vi "ENACreateMeas.vi"(0 "Meas in":T1={"S11"=TRUE, "S12"=TRUE, "S21"=TRUE, "S22"=TRUE}) -> (1 "Meas parameters":u16[](array[ring]) items=["S11", "S21", "S31", "S41", "S12", "S22", "S32", "S42", "S13", "S23", "S33", "S43", "S14", "S24", "S34", "S44", "A", "B", "C", "D", "R1", "R2", "R3", "R4", "AUX1", "AUX2", "TR", "T", "R"], 2 "Data format":u16[](array[ring]) items=["Logarithmic Magnitude", "Phase", "Group Delay", "Smith Chart  Linear (Lin/Phase)", "Smith Chart  Logarithmic (Log/Phase)", "Smith Chart  Complex (Real/Imag)", "Smith Chart  Impedance (R+jX)", "Smith Chart  Admittance (G+jB)", "Polar Format (Linear)", "Polar Format (Logarithmic)", "Polar Format (Re/Im)", "Linear Magnitude", "SWR", "Real", "Imaginary", "Epanded Phase", "Positive Phase"], 3 "Active trace":i32[](array[numeric]))   [LabVIEW 2017]
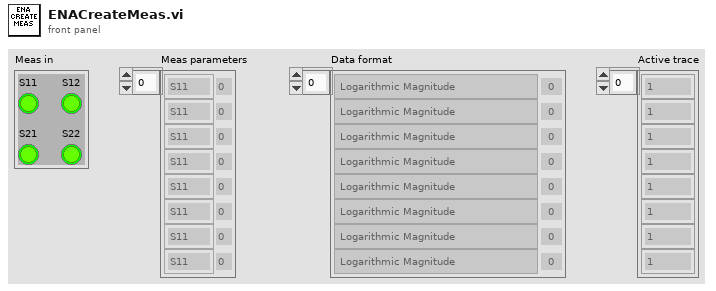
[diagram p1: front panel]
types:
  T1 = cluster{"S11":bool, "S12":bool, "S21":bool, "S22":bool}
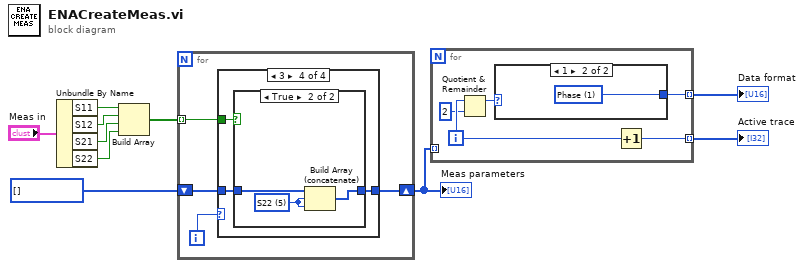
[diagram p0: block diagram]
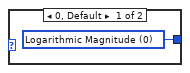
[diagram p2: hidden frame]
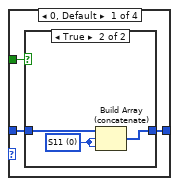
[diagram p3: hidden frame]
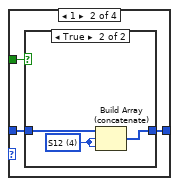
[diagram p5: hidden frame]
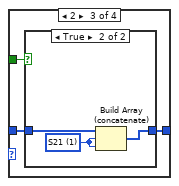
[diagram p7: hidden frame]
diagram:
  w4 = u16[] [] items=["S11", "S21", "S31", "S41", "S12", "S22", "S32", "S42", "S13", "S23", "S33", "S43", "S14", "S24", "S34", "S44", "A", "B", "C", "D", "R1", "R2", "R3", "R4", "AUX1", "AUX2", "TR", "T", "R"] ("Meas parameters 2")
  n1 = Unbundle By Name("Meas in") -> ("S11"=w9:bool, "S12"=w8:bool, "S21"=w7:bool, "S22"=w6:bool)
  n2 = Build Array(w9, w8, w7, w6) -> (w5:bool[])
  n3 = for {
    tunnel: w5 -> [w14] mode=indexing
    shift-right: [w11] -> w3
    shift-left: w4 -> [w13]
    i -> [w12]
    n4 = case shown="3" w12 {
      tunnel: w14 -> [w17 w24 w31 w38]
      tunnel: w13 -> [w16 w23 w30 w37]
      tunnel: [w15 w22 w29 w36] -> w11
      frame 0, Default {
        n5 = case shown="True" w17 {
          tunnel: w16 -> [w18 w20]
          tunnel: [w18 w21] -> w15
          frame False {
          }
          frame True {
            w19 = u16 0 items=["S11", "S21", "S31", "S41", "S12", "S22", "S32", "S42", "S13", "S23", "S33", "S43", "S14", "S24", "S34", "S44", "A", "B", "C", "D", "R1", "R2", "R3", "R4", "AUX1", "AUX2", "TR", "T", "R"] ("Measurement Parameters (0: S11)")
            n6 = Build Array (concatenate)(w20, w19, w19) -> (w21:u16[])
          }
        }
      }
      frame 1 {
        n7 = case shown="True" w24 {
          tunnel: w23 -> [w25 w27]
          tunnel: [w25 w28] -> w22
          frame False {
          }
          frame True {
            w26 = u16 4 items=["S11", "S21", "S31", "S41", "S12", "S22", "S32", "S42", "S13", "S23", "S33", "S43", "S14", "S24", "S34", "S44", "A", "B", "C", "D", "R1", "R2", "R3", "R4", "AUX1", "AUX2", "TR", "T", "R"] ("Measurement Parameters (0: S11)")
            n8 = Build Array (concatenate)(w27, w26, w26) -> (w28:u16[])
          }
        }
      }
      frame 2 {
        n9 = case shown="True" w31 {
          tunnel: w30 -> [w32 w34]
          tunnel: [w32 w35] -> w29
          frame False {
          }
          frame True {
            w33 = u16 1 items=["S11", "S21", "S31", "S41", "S12", "S22", "S32", "S42", "S13", "S23", "S33", "S43", "S14", "S24", "S34", "S44", "A", "B", "C", "D", "R1", "R2", "R3", "R4", "AUX1", "AUX2", "TR", "T", "R"] ("Measurement Parameters (0: S11)")
            n10 = Build Array (concatenate)(w34, w33, w33) -> (w35:u16[])
          }
        }
      }
      frame 3 {
        n11 = case shown="True" w38 {
          tunnel: w37 -> [w39 w41]
          tunnel: [w39 w42] -> w36
          frame False {
          }
          frame True {
            w40 = u16 5 items=["S11", "S21", "S31", "S41", "S12", "S22", "S32", "S42", "S13", "S23", "S33", "S43", "S14", "S24", "S34", "S44", "A", "B", "C", "D", "R1", "R2", "R3", "R4", "AUX1", "AUX2", "TR", "T", "R"] ("Measurement Parameters (0: S11)")
            n12 = Build Array (concatenate)(w41, w40, w40) -> (w42:u16[])
          }
        }
      }
    }
  }
  "Meas parameters" <- w3
  n13 = for {
    tunnel: w3 -> [_] mode=indexing
    tunnel: [w47] -> w2 mode=indexing
    tunnel: [w46] -> w1 mode=indexing
    i -> [w45]
    n14 = Quotient & Remainder(x=w45, y=2) -> (x-y*floor(x/y)=w43:i32)  [unwired: 1 out]
    n15 = case shown="1" w43 {
      tunnel: [w48 w49] -> w46
      frame 0, Default {
        w48 = u16 0 items=["Logarithmic Magnitude", "Phase", "Group Delay", "Smith Chart  Linear (Lin/Phase)", "Smith Chart  Logarithmic (Log/Phase)", "Smith Chart  Complex (Real/Imag)", "Smith Chart  Impedance (R+jX)", "Smith Chart  Admittance (G+jB)", "Polar Format (Linear)", "Polar Format (Logarithmic)", "Polar Format (Re/Im)", "Linear Magnitude", "SWR", "Real", "Imaginary", "Epanded Phase", "Positive Phase"] ("Data Format (0: Logarithmic Magnitude)")
      }
      frame 1 {
        w49 = u16 1 items=["Logarithmic Magnitude", "Phase", "Group Delay", "Smith Chart  Linear (Lin/Phase)", "Smith Chart  Logarithmic (Log/Phase)", "Smith Chart  Complex (Real/Imag)", "Smith Chart  Impedance (R+jX)", "Smith Chart  Admittance (G+jB)", "Polar Format (Linear)", "Polar Format (Logarithmic)", "Polar Format (Re/Im)", "Linear Magnitude", "SWR", "Real", "Imaginary", "Epanded Phase", "Positive Phase"] ("Data Format (0: Logarithmic Magnitude)")
      }
    }
    n16 = Increment(x=w45) -> (x+1=w47:i32)
  }
  "Data format" <- w1
  "Active trace" <- w2
